vi "Set Buffer.vi"(6 "Set? [T]":bool=TRUE, 7 "Config in":refnum<class "Carya Config.lvclass">, 8 "error in (no error)":errorcluster, 11 "Carya Config (Buffer) in":refnum<class "CConfig By Ref Buffer.lvclass">) -> (0 "error out":errorcluster, 2 "Replace?":bool=TRUE, 3 "Carya Config (Buffer) out":refnum<class "CConfig By Ref Buffer.lvclass">)   [LabVIEW 2013, in "CConfig By Ref Buffer.lvclass"]
doc: "Copyright 2018, Carya Automatisering, Wiebe Walstra."
uses:
  CConfig By Ref Buffer.lvclass
  Carya Config.lvclass
  Buffer Functions.ctl
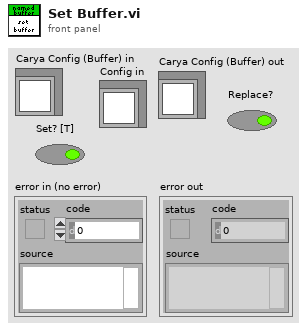
[diagram p1: front panel]
types:
  T1 = typedef "CConfig By Ref Buffer.lvclass/Buffer Functions.ctl" = enum16{"register", "get and lock", "set and unlock", "unlock", "unregister", "check"}
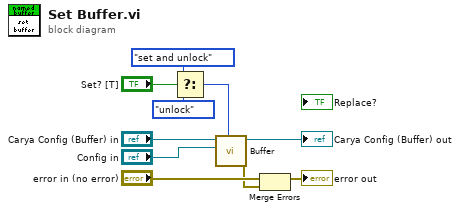
[diagram p0: block diagram]
diagram:
  n1 = Select(t=Buffer_Functions."set and unlock" ("Functions"), s="Set? [T]", f=Buffer_Functions."unlock") -> (s? t:f=w3:T1)
  n2 = call "Buffer.vi"("Functions"=w3, "Config in"="Config in", "Carya Config (Buffer) in"="Carya Config (Buffer) in") -> ("error out"=w7:errorcluster, "Carya Config (Buffer) out"=→"Carya Config (Buffer) out":refnum<class "CConfig By Ref Buffer.lvclass">)  [unwired: 4 in, 3 out]
  n3 = Merge Errors("error in (no error)", w7) -> (→"error out":errorcluster)
